vi "Autonomous Independent.vi"   [LabVIEW 2012]
doc: "This VI is called when autonomous begins, and will automatically be terminated when autonomous ends. You can carry out timed or sensor driven robot movement independently without needing to return to the caller."
uses:
  Robot Global Data.vi
  Auton Globals.vi
  Arm Globals.vi
panel:
  # "Be sure to right-click and choose Data Operations>>Make Current Value default if you want to save the array values with the VI"
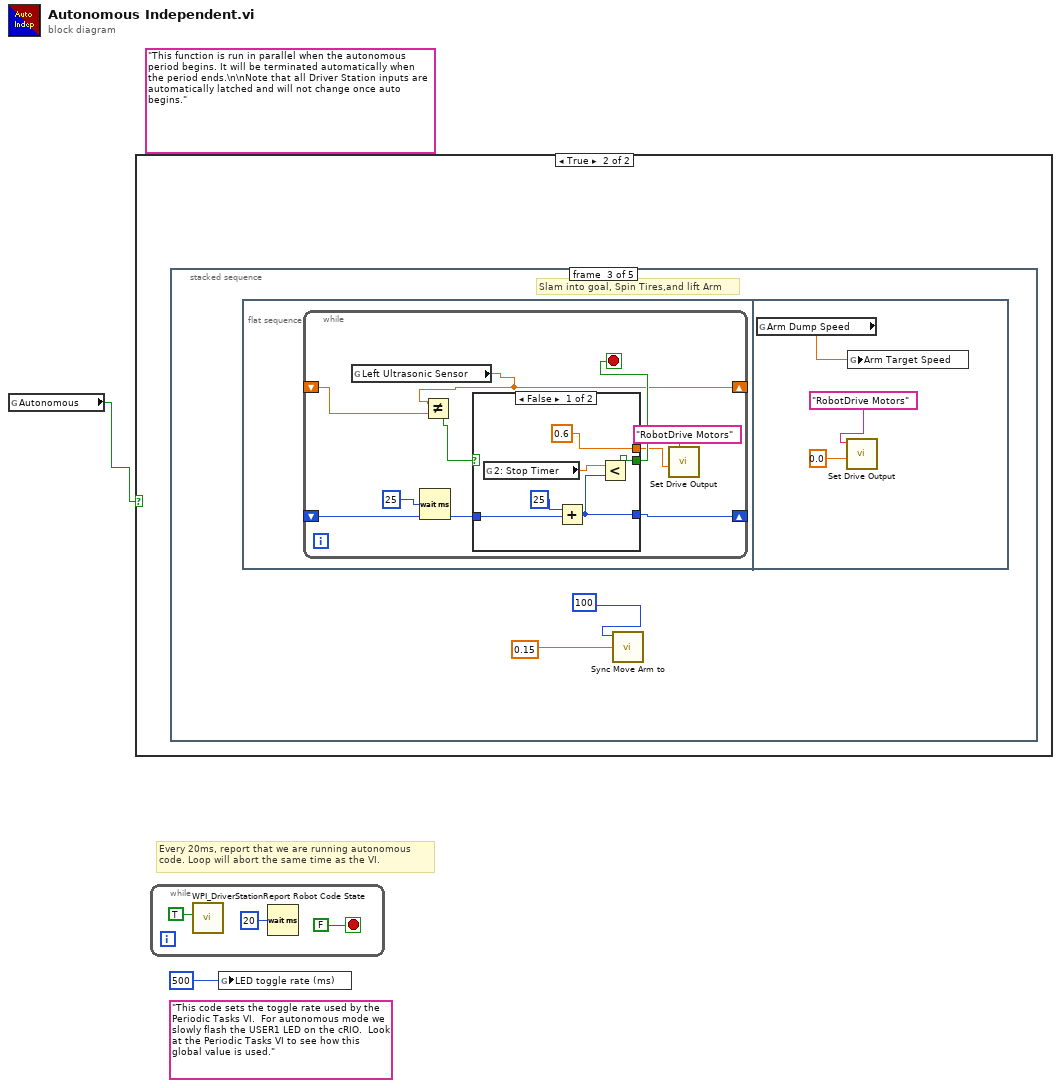
[diagram p0: block diagram]
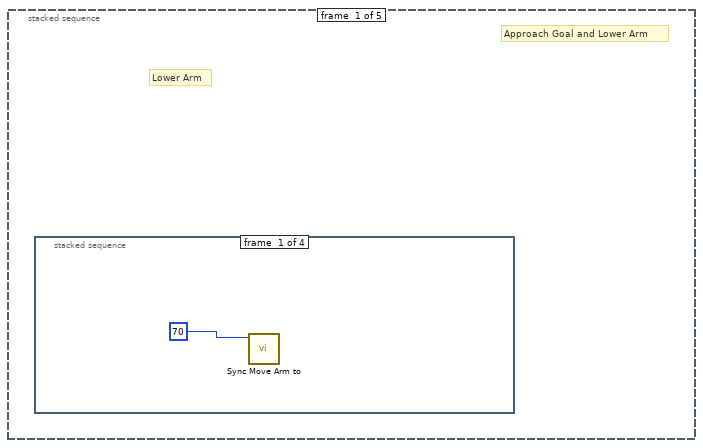
[diagram p3: hidden frame]
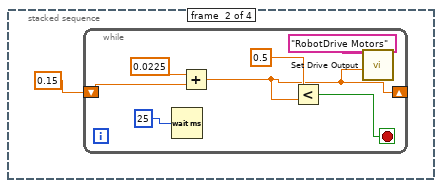
[diagram p4: hidden frame]
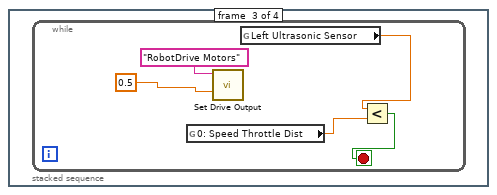
[diagram p5: hidden frame]
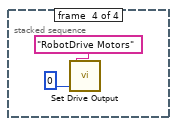
[diagram p6: hidden frame]
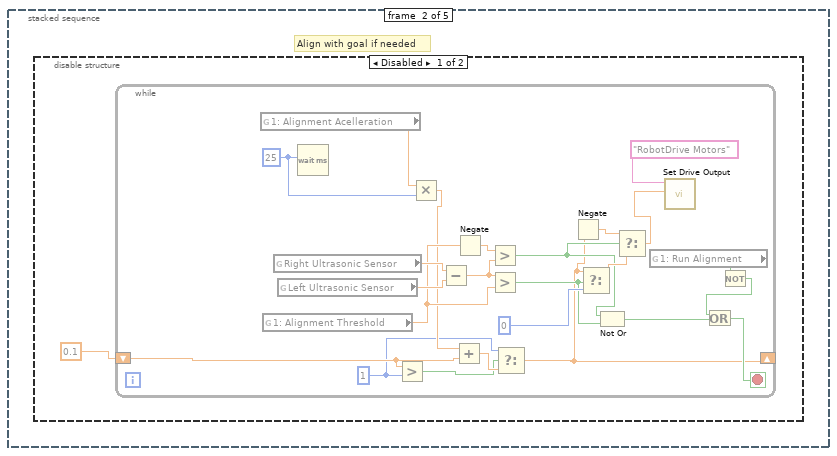
[diagram p7: hidden frame]
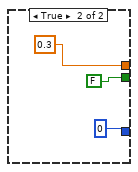
[diagram p9: hidden frame]
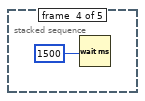
[diagram p10: hidden frame]
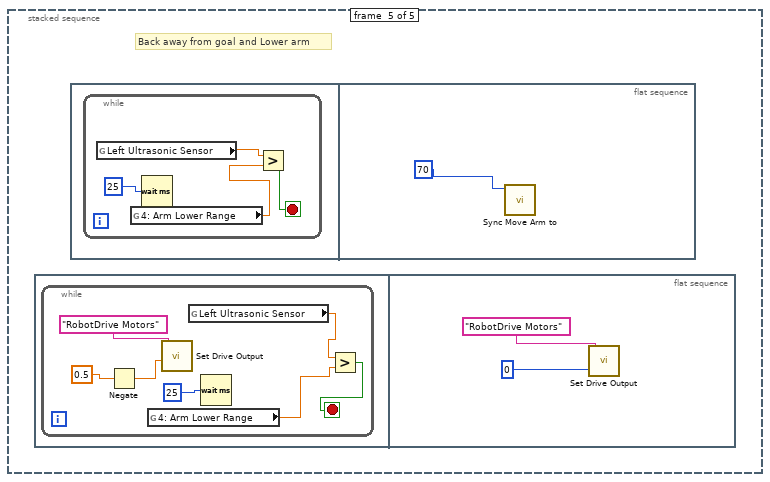
[diagram p11: hidden frame]
diagram:
  (unwired) "This code sets the toggle rate used by the Periodic Tasks VI.  For autonomous mode we slowly flash the USER1 LED on the cRIO.  Look at the Periodic Tasks VI to see how this global value is used."
  (unwired) "This function is run in parallel when the autonomous period begins. It will be terminated automatically when the period ends.\n\nNote that all Driver Station inputs are automatically latched and will not change once auto begins."
  # "Every 20ms, report that we are running autonomous\ncode. Loop will abort the same time as the VI."
  n1 = global read "Robot Global Data.vi" "Autonomous"() -> (w1:bool)
  n2 = case shown="True" w1 {
    frame False {
    }
    frame True {
      n3 = stacked-sequence {
        frame #0 {
          # "Lower Arm"
          # "Approach Goal and Lower Arm"
          n4 = stacked-sequence {
            frame #0 {
              n5 = call "Sync Move Arm to.vi"("Target Position"=70) -> ()  [unwired: 11 in]
            }
            frame #1 {
              n6 = while {
                shift-right: [w7] -> _
                shift-left: 0.15 -> [w11]
                stop <- w9 stop-if-true
                n7 = Wait (ms)(milliseconds to wait=25) -> ()  [unwired: 1 out]
                n8 = Add(x=0.0225, y=w11) -> (x+y=w7:dbl)
                n9 = Less?(x=0.5, y=w7) -> (x < y?=w9:bool)
                n10 = call "Set Drive Output.vi"("Y axis"=w7, "Drive RefNum"="RobotDrive Motors") -> ()  [unwired: 8 in]
              }
            }
            frame #2 {
              n11 = while {
                stop <- w15 stop-if-true
                n12 = global read "Auton Globals.vi" "0: Speed Throttle Dist"() -> (w14:dbl)
                n13 = call "Set Drive Output.vi"("Y axis"=0.5, "Drive RefNum"="RobotDrive Motors") -> ()  [unwired: 8 in]
                n14 = global read "Robot Global Data.vi" "Left Ultrasonic Sensor"() -> (w13:dbl)
                n15 = Less?(x=w13, y=w14) -> (x < y?=w15:bool)
              }
            }
            frame #3 {
              n16 = call "Set Drive Output.vi"("Y axis"=0, "Drive RefNum"="RobotDrive Motors") -> ()  [unwired: 8 in]
            }
          }
        }
        frame #1 {
          # "Align with goal if needed"
          n17 = disable-structure shown="Disabled" {
            frame Disabled {
              n18 = while {
                shift-right: [w20] -> _
                shift-left: 0.1 -> [w24]
                stop <- w41 stop-if-true
                w21 = 1
                w28 = 25
                n19 = global read "Auton Globals.vi" "1: Alignment Acelleration"() -> (w29:dbl)
                n20 = global read "Auton Globals.vi" "1: Alignment Threshold"() -> (w36:dbl)
                n21 = global read "Robot Global Data.vi" "Right Ultrasonic Sensor"() -> (w40:dbl)
                n22 = global read "Robot Global Data.vi" "Left Ultrasonic Sensor"() -> (w39:dbl)
                n23 = Wait (ms)(milliseconds to wait=w28) -> ()  [unwired: 1 out]
                n24 = Greater?(x=w24, y=w21) -> (0:w22:bool)
                n25 = Multiply(x=w29, y=w28) -> (x*y=w27:dbl)
                n26 = Subtract(x=w40, y=w39) -> (x-y=w38:dbl)
                n27 = Add(x=w27, y=w24) -> (x+y=w23:dbl)
                n28 = Negate(x=w36) -> (-x=w37:dbl)
                n29 = Greater?(x=w37, y=w38) -> (0:w33:bool)
                n30 = Greater?(x=w38, y=w36) -> (0:w32:bool)
                n31 = Select(t=w21, s=w22, f=w23) -> (s? t:f=w20:dbl)
                n32 = Negate(x=w20) -> (-x=w30:dbl)
                n33 = Select(t=w20, s=w32, f=0) -> (s? t:f=w35:dbl)
                n34 = Not Or(1:w32, 2:w33) -> (0:w31:bool)
                n35 = Select(t=w30, s=w33, f=w35) -> (s? t:f=w25:dbl)
                n36 = global read "Auton Globals.vi" "1: Run Alignment"() -> (w43:bool)
                n37 = call "Set Drive Output.vi"("X axis"=w25, "Drive RefNum"="RobotDrive Motors" ("Name")) -> ()  [unwired: 8 in]
                n38 = Not(x=w43) -> (.not. x?=w42:bool)
                n39 = Or(x=w42, y=w31) -> (x .or. y?=w41:bool)
              }
            }
            frame Enabled {
            }
          }
        }
        frame #2 {
          # "Slam into goal, Spin Tires,and lift Arm"
          n40 = flat-sequence {
            frame #0 {
              n41 = while {
                shift-right: [w52] -> _
                shift-left: _ -> [w51]
                shift-right: [w47] -> _
                shift-left: _ -> [w48]
                stop <- w49 stop-if-true
                n42 = global read "Robot Global Data.vi" "Left Ultrasonic Sensor"() -> (w47:dbl)
                n43 = Wait (ms)(milliseconds to wait=25) -> ()  [unwired: 1 out]
                n44 = Not Equal?(x=w47, y=w48) -> (x != y?=w50:bool)
                n45 = case shown="False" w50 {
                  tunnel: [w57 FALSE] -> w49
                  tunnel: [w58 0] -> w52
                  tunnel: w51 -> [w60 _]
                  tunnel: [0.6 0.3] -> w46
                  frame False {
                    n46 = global read "Auton Globals.vi" "2: Stop Timer"() -> (w56:dbl)
                    n47 = Add(x=25, y=w60) -> (x+y=w58:i32)
                    n48 = Less?(x=w56, y=w58) -> (x < y?=w57:bool)
                  }
                  frame True {
                  }
                }
                n49 = call "Set Drive Output.vi"("Y axis"=w46, "Drive RefNum"="RobotDrive Motors") -> ()  [unwired: 8 in]
              }
            }
            frame #1 {
              n50 = global read "Arm Globals.vi" "Arm Dump Speed"() -> (w64:dbl)
              n51 = call "Set Drive Output.vi"("Y axis"=0.0, "Drive RefNum"="RobotDrive Motors") -> ()  [unwired: 8 in]
              n52 = global write "Robot Global Data.vi" "Arm Target Speed"(w64) -> ()
            }
          }
          n53 = call "Sync Move Arm to.vi"("Speed"=0.15, "Target Position"=100) -> ()  [unwired: 10 in]
        }
        frame #3 {
          n54 = Wait (ms)(milliseconds to wait=1500) -> ()  [unwired: 1 out]
        }
        frame #4 {
          # "Back away from goal and Lower arm"
          n55 = flat-sequence {
            frame #0 {
              n56 = while {
                stop <- w78 stop-if-true
                n57 = Negate(x=0.5) -> (-x=w75:dbl)
                n58 = global read "Auton Globals.vi" "4: Arm Lower Range"() -> (w76:dbl)
                n59 = call "Set Drive Output.vi"("Y axis"=w75, "Drive RefNum"="RobotDrive Motors") -> ()  [unwired: 8 in]
                n60 = global read "Robot Global Data.vi" "Left Ultrasonic Sensor"() -> (w74:dbl)
                n61 = Wait (ms)(milliseconds to wait=25) -> ()  [unwired: 1 out]
                n62 = Greater?(x=w74, y=w76) -> (0:w78:bool)
              }
            }
            frame #1 {
              n63 = call "Set Drive Output.vi"("Y axis"=0, "Drive RefNum"="RobotDrive Motors") -> ()  [unwired: 8 in]
            }
          }
          n64 = flat-sequence {
            frame #0 {
              n65 = while {
                stop <- w71 stop-if-true
                n66 = global read "Robot Global Data.vi" "Left Ultrasonic Sensor"() -> (w68:dbl)
                n67 = global read "Auton Globals.vi" "4: Arm Lower Range"() -> (w69:dbl)
                n68 = Wait (ms)(milliseconds to wait=25) -> ()  [unwired: 1 out]
                n69 = Greater?(x=w68, y=w69) -> (0:w71:bool)
              }
            }
            frame #1 {
              n70 = call "Sync Move Arm to.vi"("Target Position"=70) -> ()  [unwired: 11 in]
            }
          }
        }
      }
    }
  }
  n71 = while {
    stop <- FALSE stop-if-true
    n72 = call <vilib>:"WPI_DriverStationReport Robot Code State.vi"("Autonomous"=TRUE) -> ()  [unwired: 10 in, 1 out]
    n73 = Wait (ms)(milliseconds to wait=u32 20) -> ()  [unwired: 1 out]
  }
  n74 = global write "Robot Global Data.vi" "LED toggle rate (ms)"(u32 500 ("LED ms toggle rate")) -> ()
